vi "Write Hold plot upper.vi"(8 "error in (no error)":errorcluster, 10 "Hold plot upper":bool caption="Hold plot", 11 "Scope5761":refnum<class "Scope5782_six_channel.lvclass">) -> (0 "error out":errorcluster, 3 "Scope5761":refnum<class "Scope5782_six_channel.lvclass">)   [LabVIEW 2018, in "Scope5782_six_channel.lvclass"]
uses:
  Scope5782_six_channel.lvclass
  Scope5782_six_channel.lvclass/Scope5782_six_channel.ctl
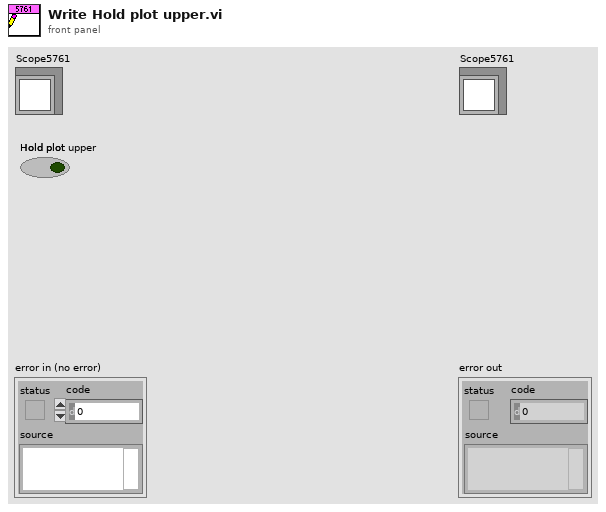
[diagram p1: front panel]
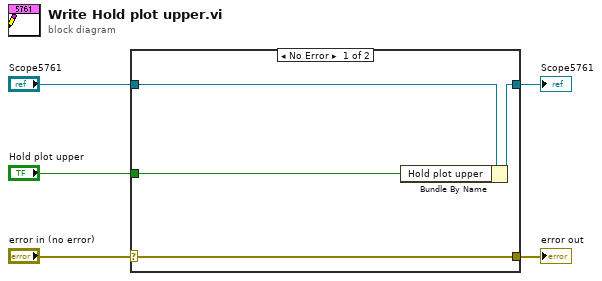
[diagram p0: block diagram]
diagram:
  n1 = case shown="No Error" "error in (no error)" {
    selector: "error in (no error)" -> [w9 w10]
    tunnel: [w9 w10] -> w4
    tunnel: [w7 w11] -> w2
    tunnel: "Scope5761" -> [w8 w11]
    tunnel: "Hold plot upper" -> [w6 _]
    frame No Error {
      n2 = Bundle By Name(cluster=w8, "Hold plot upper"=w6) -> (w7:refnum<class "Scope5782_six_channel.lvclass">)
    }
    frame Error {
    }
  }
  "error out" <- w4
  "Scope5761" <- w2
